vi "Clear infused_withdrawn Volume.vi"(8 "error in (no error)":errorcluster, 11 "VISA resource name":refnum<visa-resource-name>) -> (0 "error out":errorcluster, 3 "VISA resource name out":refnum<visa-resource-name>)   [LabVIEW 2016]
panel:
  in  "VISA wait (msec)":u32=100
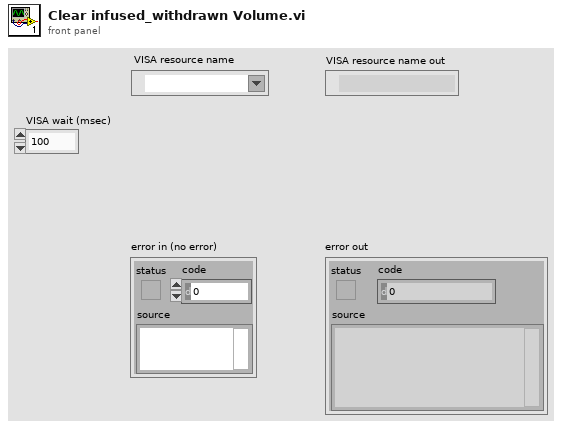
[diagram p1: front panel]
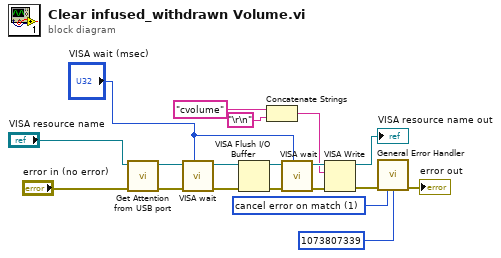
[diagram p0: block diagram]
diagram:
  w8 = 1 items=["no exception", "cancel error on match", "set error on match"] ("[exception action] (none:0)")
  n1 = call "Get Attention from USB port.vi"("error in (no error)"="error in (no error)", "VISA resource name"="VISA resource name") -> ("error out"=w12:errorcluster, "VISA resource name out"=w13:refnum<visa-resource-name>)  [unwired: 8 in]
  n2 = call <userlib>:"VISA wait.vi"("VISA resource name"=w13, "error in (no error)"=w12, "milliseconds to wait"="VISA wait (msec)") -> ("VISA resource name out"=w11:refnum<visa-resource-name>, "error out"=w10:errorcluster)  [unwired: 6 in]
  n3 = VISA Flush I/O Buffer(VISA resource name=w11, error in (no error)=w10) -> (VISA resource name out=w17:refnum<visa-resource-name>, error out=w16:errorcluster)  [unwired: 1 in]
  n4 = Concatenate Strings("cvolume" ("multi-line string"), "\r\n") -> (w4:string)
  n5 = call <userlib>:"VISA wait.vi"("VISA resource name"=w17, "error in (no error)"=w16, "milliseconds to wait"="VISA wait (msec)") -> ("VISA resource name out"=w15:refnum<visa-resource-name>, "error out"=w14:errorcluster)  [unwired: 6 in]
  n6 = VISA Write(VISA resource name=w15, write buffer=w4, error in (no error)=w14) -> (VISA resource name out=→"VISA resource name out":refnum<visa-resource-name>, error out=w1:errorcluster)  [unwired: 1 out]
  n7 = call <vilib>:"General Error Handler.vi"("error in (no error)"=w1, "[exception action] (none:0)"=w8, "[exception code]"=1073807339) -> ("error out"=→"error out":errorcluster)  [unwired: 8 in, 4 out]
